vi "VerifyArguments.vi"(8 "error in (no error)":errorcluster, 11 "ExecuteMultipleBuildSpecs in":refnum<class "ExecuteMultipleBuildSpecs.lvclass">) -> (0 "error out":errorcluster, 3 "ExecuteMultipleBuildSpecs out":refnum<class "ExecuteMultipleBuildSpecs.lvclass">)   [LabVIEW 2022 SP3, in "ExecuteMultipleBuildSpecs.lvclass"]
doc: "Ensures required arguments are provided to the LabVIEWCLI."
uses:
  ExecuteMultipleBuildSpecs.lvclass
  ExecuteMultipleBuildSpecs.lvclass/ExecuteMultipleBuildSpecs.ctl
  Program Files (x86)/National Instruments/Shared/LabVIEW CLI/Operations/Utilities/OperationErrorType.ctl
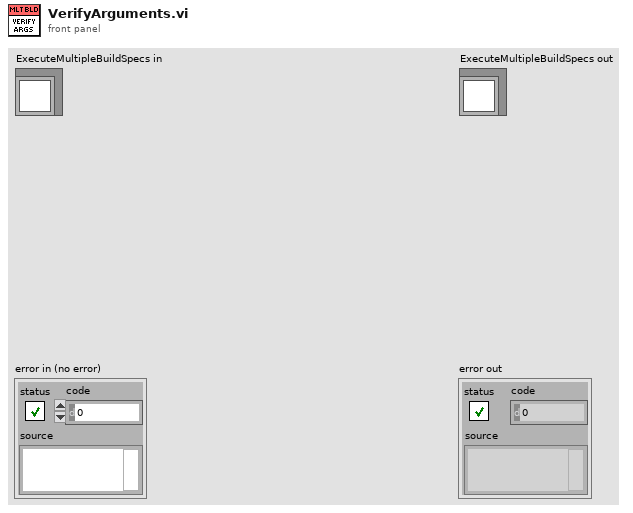
[diagram p1: front panel]
types:
  T1 = typedef "OperationErrorType.ctl" = enum16{"RequiredArgumentMissing", "UnknownArguments", "LoggerSetMultipleTimes", "OperationBrokenError"}
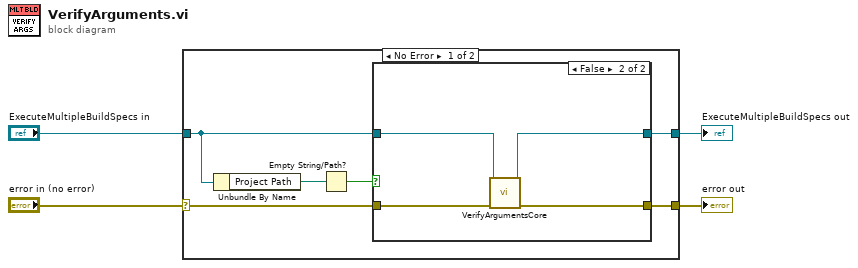
[diagram p0: block diagram]
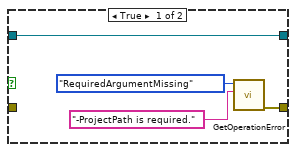
[diagram p2: hidden frame]
diagram:
  n1 = case shown="No Error" "error in (no error)" {
    selector: "error in (no error)" -> [w6 w20]
    tunnel: [w5 w20] -> w3
    tunnel: [w7 w19] -> w1
    tunnel: "ExecuteMultipleBuildSpecs in" -> [w8 w19]
    frame No Error {
      n2 = Unbundle By Name(w8) -> ("Project Path"=w9:path)
      n3 = Empty String/Path?(string/path=w9) -> (empty?=w10:bool)
      n4 = case shown="False" w10 {
        tunnel: w6 -> [_ w18]
        tunnel: [w13 w17] -> w5
        tunnel: w8 -> [w14 w16]
        tunnel: [w14 w15] -> w7
        frame True {
          n5 = call "GetOperationError.vi"("Additional Information"="-ProjectPath is required.", "Operation Error Type"=OperationErrorType."RequiredArgumentMissing") -> ("error out"=w13:errorcluster)  [unwired: 9 in]
        }
        frame False {
          n6 = call-dynamic "VerifyArgumentsCore.vi"("error in (no error)"=w18, "ExecuteMultipleBuildSpecs in"=w16) -> ("error out"=w17:errorcluster, "ExecuteMultipleBuildSpecs out"=w15:refnum<class "ExecuteMultipleBuildSpecs.lvclass">)  [unwired: 8 in]
        }
      }
    }
    frame Error {
    }
  }
  "error out" <- w3
  "ExecuteMultipleBuildSpecs out" <- w1
